vi "柱塞泵组合启动命令.vi"(8 "Error in":errorcluster caption="Error in (no error)", 11 "仪器":enum16{"", "氨氮", "总磷", "总氮", "CODMn", "CODCr"}(ring)=enum."氨氮") -> (0 "error out":errorcluster)   [LabVIEW 2016, in "质控单元.lvlib"]
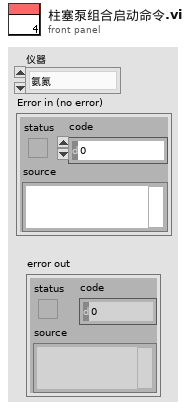
[diagram p1: front panel]
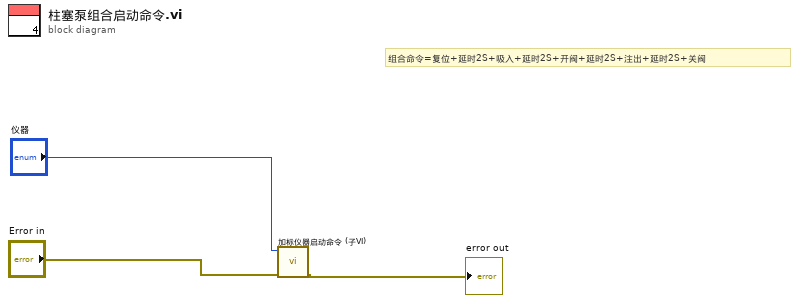
[diagram p0: block diagram]
diagram:
  # "组合命令=复位+延时2S+吸入+延时2S+开阀+延时2S+注出+延时2S+关阀"
  n1 = call "加标仪器启动命令 (子VI).vi"("错误输入（无错误）"="Error in", "仪器"="仪器") -> ("错误输出"=→"error out":errorcluster)  [unwired: 9 in]
